vi "ColorJudge.vi"(1 "B":u8, 2 "G":u8, 3 "R":u8, 4 "C":u32(colorbox)) -> (0 "out":bool)   [LabVIEW 2017]
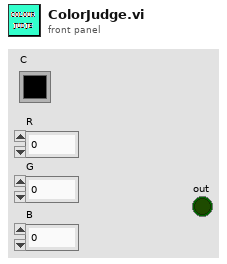
[diagram p1: front panel]
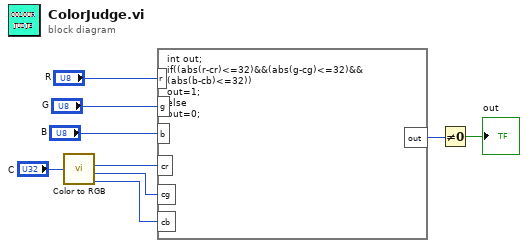
[diagram p0: block diagram]
diagram:
  n1 = call <vilib>:"Color to RGB.vi"("Color"="C") -> ("R"=w5:u8, "G"=w4:u8, "B"=w3:u8)  [unwired: 1 out]
  n2 = formula code="int out;\nif((abs(r-cr)<=32)&&(abs(g-cg)<=32)&&\n(abs(b-cb)<=32))\nout=1;\nelse\nout=0;"("r"="R", "g"="G", "b"="B", "cr"=w5, "cg"=w4, "cb"=w3) -> ("out"=w2:i32)
  n3 = Not Equal To 0?(x=w2) -> (x != 0?=→"out":bool)
